vi "IR sensors.vi"(8 "error in":errorcluster, 11 "FPGA VI Reference In":refnum<k20>) -> (0 "error out":errorcluster, 2 "IR Sensors":dbl[](array[numeric]), 3 "FPGA VI Reference Out":refnum<k20>)   [LabVIEW 2019]
uses:
  <vilib>/Utility/error.llb/Error Cluster From Error Code.vi
  <vilib>/rvi/errors/niLvFpgaAdjustHostInterfaceError.vi
  <vilib>/rvi/interface/nirviReadWriteControl/nirviReadWriteControl.xnode
  NiFpgaLv.dll
  <vilib>/rvi/interface/Simulation/niFpgaSimulationCallBeginRW.vi
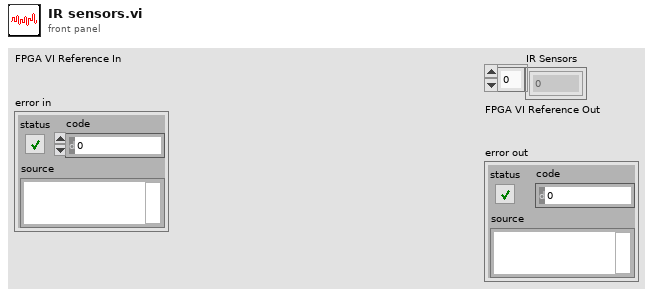
[diagram p1: front panel]
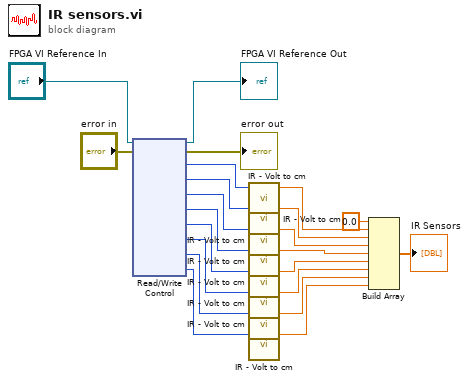
[diagram p0: block diagram]
diagram:
  n1 = xnode "Read/Write Control"("FPGA VI Reference In"="FPGA VI Reference In", "error in"="error in") -> ("FPGA VI Reference Out"=→"FPGA VI Reference Out":refnum<k20>, "error out"=→"error out":errorcluster, "IR 1"=w22:u16, "IR 2"=w16:u16, "IR 3"=w15:u16, "IR 4"=w14:u16, "IR 5"=w13:u16, "IR 6"=w12:u16, "IR 7"=w11:u16, "IR 8"=w10:u16)
  n2 = call "IR - Volt to cm.vi"("Volt"=w22) -> ("Distance (cm)"=w2:dbl)  [unwired: 4 in]
  n3 = call "IR - Volt to cm.vi"("Volt"=w16) -> ("Distance (cm)"=w3:dbl)  [unwired: 4 in]
  n4 = call "IR - Volt to cm.vi"("Volt"=w15) -> ("Distance (cm)"=w4:dbl)  [unwired: 4 in]
  n5 = call "IR - Volt to cm.vi"("Volt"=w14) -> ("Distance (cm)"=w5:dbl)  [unwired: 4 in]
  n6 = call "IR - Volt to cm.vi"("Volt"=w13) -> ("Distance (cm)"=w6:dbl)  [unwired: 4 in]
  n7 = call "IR - Volt to cm.vi"("Volt"=w12) -> ("Distance (cm)"=w7:dbl)  [unwired: 4 in]
  n8 = call "IR - Volt to cm.vi"("Volt"=w11) -> ("Distance (cm)"=w8:dbl)  [unwired: 4 in]
  n9 = call "IR - Volt to cm.vi"("Volt"=w10) -> ("Distance (cm)"=w9:dbl)  [unwired: 4 in]
  n10 = Build Array(0.0 ("element"), w2, w3, w4, w5, w6, w7, w8, w9) -> (→"IR Sensors":dbl[])
